vi "newmark_open.vi"(8 "error in":errorcluster, 11 "VISA Refnum in":refnum<visa-resource-name>="COM1") -> (0 "error out":errorcluster, 3 "VISA Refnum out":refnum<visa-resource-name>)   [LabVIEW 2011]
uses:
  <vilib>/Instr/_visa.llb/VISA Configure Serial Port (Instr).vi
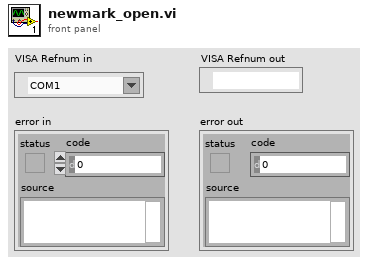
[diagram p1: front panel]
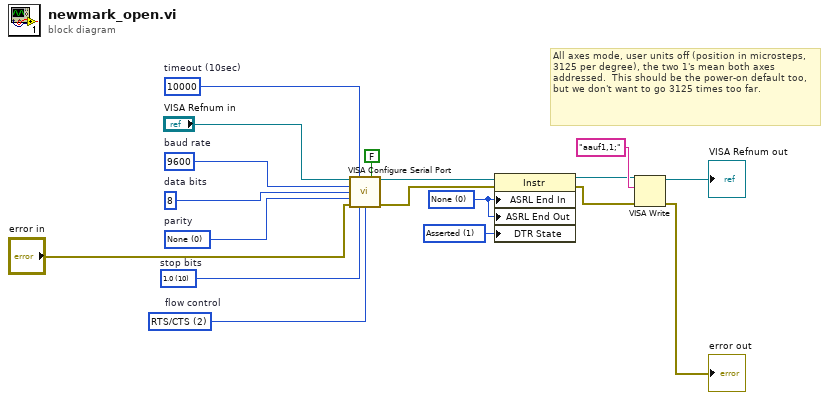
[diagram p0: block diagram]
diagram:
  w1 = i16 1 items=["Unknown"=-1, "Unasserted"=0, "Asserted"=1] ("Serial Settings:Modem Line Settings:Line DTR State")
  w5 = u16 0 items=["None", "Last Bit", "TermChar"] ("Serial Settings:End Mode for Reads")
  w16 = u16 2 items=["None"=0, "XON/XOFF"=1, "RTS/CTS"=2, "DTR/DSR"=4]  # flow control
  w15 = u16 10 items=["1.0"=10, "1.5"=15, "2.0"=20]  # stop bits
  w13 = u16 0 items=["None", "Odd", "Even", "Mark", "Space"]  # parity
  w17 = u16 8  # data bits
  w11 = u32 9600  # baud rate
  w14 = u32 10000  # timeout (10sec)
  # "All axes mode, user units off (position in microsteps, 3125 per degree), the two 1's mean both axes addressed.  This should be the power-on default too, but we don't want to go 3125 times too far."
  n1 = call-poly "VISA Configure Serial Port"("VISA resource name"="VISA Refnum in", "timeout (10sec)"=w14, "Enable Termination\nChar (T)"=FALSE ("Enable Termination\nChar (T)"), "baud rate (9600)"=w11, "data bits (8)"=w17, "parity (0:none)"=w13, "error in (no error)"="error in", "stop bits (10: 1 bit)"=w15, "flow control (0:none)"=w16) -> ("VISA resource name out"=w7:refnum<visa-resource-name>, "error out"=w6:errorcluster)  [unwired: 5 out]
  n2 = property class="Instr"(reference=w7, error in=w6, "ASRL End In"=w5, "ASRL End Out"=w5, "DTR State"=w1) -> (reference out=w4:refnum<visa-resource-name>, error out=w3:errorcluster)
  n3 = VISA Write(VISA resource name=w4, write buffer="aauf1,1;", error in (no error)=w3) -> (VISA resource name out=→"VISA Refnum out":refnum<visa-resource-name>, error out=→"error out":errorcluster)  [unwired: 1 out]
